vi "Set Header.vi"(8 "error in (no error)":errorcluster, 9 "Value":string, 10 "Header":string, 11 "Response in":refnum<class "Response.lvclass">) -> (0 "error out":errorcluster, 1 "Replaced?":bool, 3 "Response out":refnum<class "Response.lvclass">)   [LabVIEW 2023, in "Response.lvclass"]
uses:
  Response.lvclass
  Response.lvclass/Response.ctl
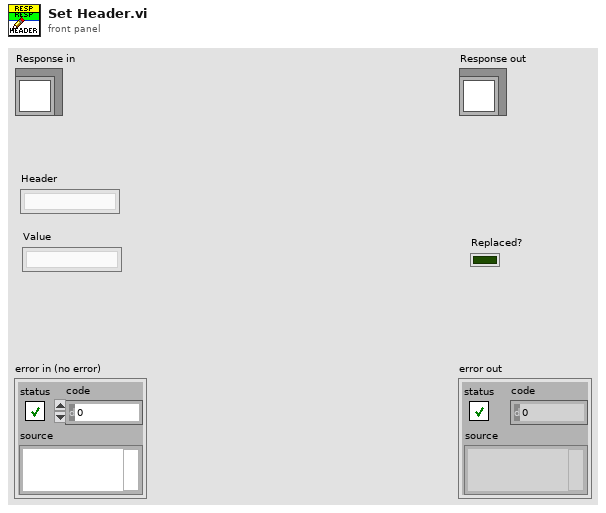
[diagram p1: front panel]
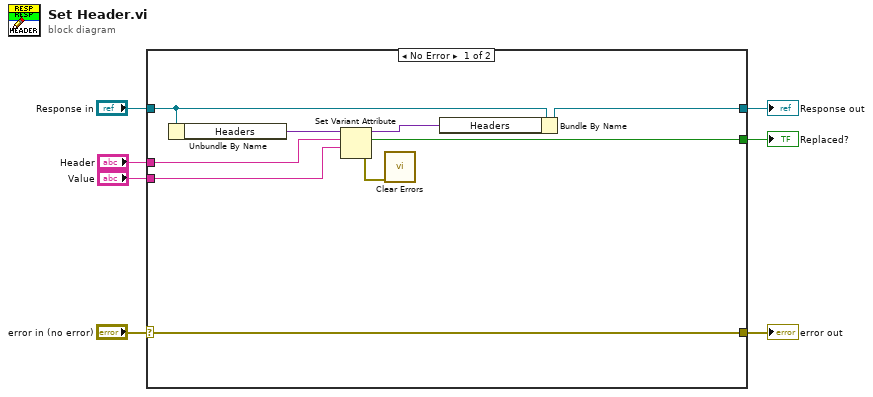
[diagram p0: block diagram]
diagram:
  n1 = case shown="No Error" "error in (no error)" {
    selector: "error in (no error)" -> [w16 w18]
    tunnel: [w16 w18] -> w6
    tunnel: [w9 w17] -> w4
    tunnel: "Response in" -> [w10 w17]
    tunnel: "Header" -> [w14 _]
    tunnel: [w12 _] -> w2
    tunnel: "Value" -> [w8 _]
    frame No Error {
      n2 = Unbundle By Name(w10) -> ("Headers"=w15:variant)
      n3 = Set Variant Attribute(Variant=w15, name=w14, value=w8) -> (Variant out=w11:variant, replaced=w12:bool, error out=w13:errorcluster)  [unwired: 1 in]
      n4 = call <vilib>:"Clear Errors.vi"("error in (no error)"=w13) -> ()  [unwired: 5 in, 2 out]
      n5 = Bundle By Name(cluster=w10, "Headers"=w11) -> (w9:refnum<class "Response.lvclass">)
    }
    frame Error {
    }
  }
  "error out" <- w6
  "Response out" <- w4
  "Replaced?" <- w2
